vi "Shooter Control.vi"(11 "Time Delay Milli":u32) -> ()   [LabVIEW 2011]
uses:
  System Set Points and States.vi
  <vilib>/addons/control/pid/pid.llb/PID (DBL).vi
  <vilib>/addons/control/pid/NI_PID_pid.lvlib
panel:
  out "Stable":bool
  out "RPM Error":cluster{dbl, dbl, dbl[]}(graph)
  out "Output 2":dbl
  out "Output":dbl
  out "Shooter Enabled":bool
  in  "Graph time interval  in seconds":dbl
  out "Shooter RPM":cluster{dbl, dbl, dbl[]}(graph)
  out "RPM Error":dbl
  out "Encoder Speed":dbl
  in  "D":dbl
  in  "I":dbl=0.0068
  in  "P":dbl=0.0017 step=0.001
  out "Encoder Set Speed":dbl
  # "These Work\n0.0045\n0.05\n0.0005"
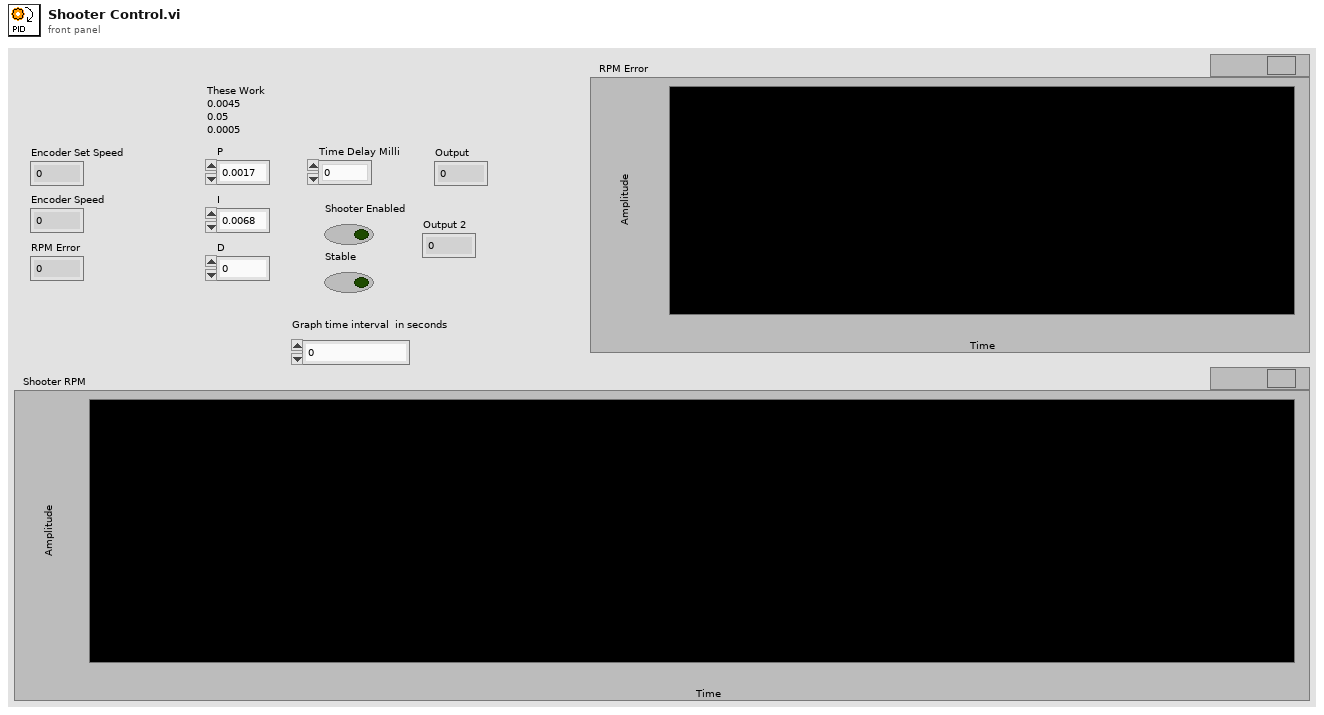
[diagram p1: front panel]
types:
  T1 = typedef "WPI_EncoderDevRef.ctl" = cluster{"DevStatus":errorcluster, "EncoderIndex":T2, "CounterIndex":T3, "DistancePerCount":dbl, "Decoding Type":T4}
  T2 = typedef "FPGA_EncoderIdx.ctl" = enum8{"Enc 0", "Enc 1", "Enc 2", "Enc 3", "Invalid"}
  T3 = typedef "FPGA_CounterCtrSystemIndex.ctl" = enum8{"Ctr 0", "Ctr 1", "Ctr 2", "Ctr 3", "Ctr 4", "Ctr 5", "Ctr 6", "Ctr 7", "Invalid"}
  T4 = typedef "WPI_EncoderType.ctl" = enum16{"1x", "2x", "4x"}
  T5 = typedef "WPI_MotorControlDeviceRef.ctl" = cluster{"DeviceStatus":errorcluster, "Type":enum16{"PWM", "CAN"}, "PWM":cluster{"Digital Module":T6, "PWM Channel":T7, "DeadBand":T8}, "CAN":cluster{"Device Number":u8, "Control Mode":T9, "Semaphore":T10, "Max Vout":dbl}, "Invert":bool, "TransformRef":T11, "InvTransformRef":T11}
  T6 = typedef "FPGA_TypedefDigitalModule.ctl" = enum16{"Digital Module 1", "Digital Module 2"}
  T7 = typedef "FPGA_DIOPWMChannel.ctl" = enum8{"PWM 1", "PWM 2", "PWM 3", "PWM 4", "PWM 5", "PWM 6", "PWM 7", "PWM 8", "PWM 9", "PWM 10", "Invalid"}
  T8 = typedef "WPI_PWMDeadband.ctl" = cluster{"Name":string, "maxPositivePwm":i32, "minPositivePwm":i32, "centerPwm":i32, "maxNegativePwm":i32, "minNegativePwm":i32, "angularRange":u16}
  T9 = typedef "WPI_CANJaguar_ControlMode.ctl" = enum8{"Percent VBus", "Current", "Speed", "Position", "Voltage"}
  T10 = typedef "Semaphore RefNum" = refnum<k1>
  T11 = typedef "WPI_PWMTransform_ConPane.ctl" = refnum<vi>
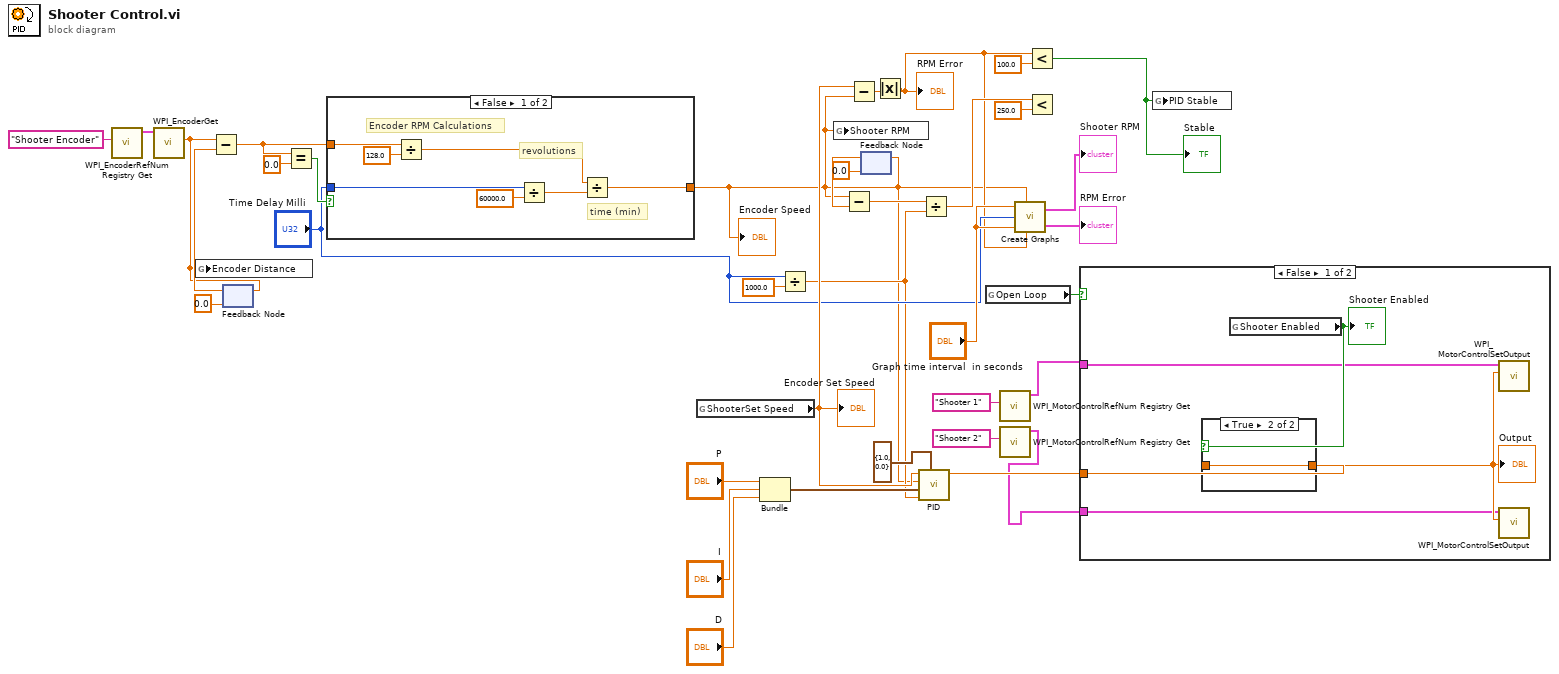
[diagram p0: block diagram]
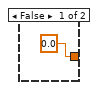
[diagram p2: hidden frame]
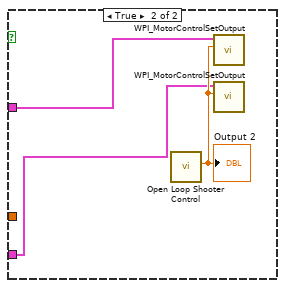
[diagram p3: hidden frame]
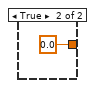
[diagram p4: hidden frame]
diagram:
  n1 = call <vilib>:"WPI_EncoderRefNum Registry Get.vi"("refnum name"="Shooter Encoder") -> ("EncoderDevRef"=w25:T1)  [unwired: 9 in, 1 out]
  n2 = call <vilib>:"WPI_EncoderGet.vi"("EncoderDevRef"=w25) -> ("Distance"=w21:dbl)  [unwired: 5 in, 5 out]
  n3 = global write "System Set Points and States.vi" "Encoder Distance"(w21) -> ()
  n4 = feedback #1(0.0) -> (w30:dbl)
  n5 = Subtract(x=w21, y=w30) -> (x-y=w22:dbl)
  n6 = feedback-in #1(w21) -> ()
  n7 = Equal?(x=w22, y=0.0) -> (x = y?=w27:bool)
  n8 = case shown="False" w27 {
    tunnel: [w43 0.0] -> w6
    tunnel: w22 -> [w42 _]
    tunnel: "Time Delay Milli" -> [w40 _]
    frame False {
      # "time (min)"
      # "revolutions"
      # "Encoder RPM Calculations"
      n9 = Divide(x=w42, y=128.0) -> (x/y=w41:dbl)
      n10 = Divide(x=w40, y=60000.0) -> (x/y=w38:dbl)
      n11 = Divide(x=w41, y=w38) -> (x/y=w43:dbl)
    }
    frame True {
    }
  }
  "Encoder Speed" <- w6
  n12 = global read "System Set Points and States.vi" "ShooterSet Speed"() -> (w31:dbl)
  "Encoder Set Speed" <- w31
  n13 = Bundle("P"="P", "I"="I", "D"="D") -> (w32:cluster{"P":dbl, "I":dbl, "D":dbl})  [unwired: 1 in]
  n14 = Divide(x="Time Delay Milli", y=1000.0) -> (x/y=w9:dbl)
  n15 = global write "System Set Points and States.vi" "Shooter RPM"(w6) -> ()
  n16 = Subtract(x=w31, y=w6) -> (x-y=w8:dbl)
  n17 = feedback-in #2(w6) -> ()
  n18 = feedback #2(0.0) -> (w20:dbl)
  n19 = Subtract(x=w6, y=w20) -> (x-y=w19:dbl)
  n20 = Absolute Value(x=w8) -> (abs(x)=w7:dbl)
  "RPM Error" <- w7
  n21 = call-poly <vilib>:"PID.vi"("output range"=cluster{"output high":dbl, "output low":dbl} {"output high"=1.0, "output low"=0.0}, "dt (s)"=w9, "PID gains"=w32, "process variable"=w6, "setpoint"=w31) -> ("output"=w24:dbl)  [unwired: 5 in, 1 out]
  n22 = Divide(x=w19, y=w9) -> (x/y=w18:dbl)
  n23 = global read "System Set Points and States.vi" "Open Loop"() -> (w23:bool)
  n24 = call <vilib>:"WPI_MotorControlRefNum Registry Get.vi"("refnum name"="Shooter 1") -> ("MotorControlDevRef"=w2:T5)  [unwired: 9 in, 1 out]
  n25 = call <vilib>:"WPI_MotorControlRefNum Registry Get.vi"("refnum name"="Shooter 2") -> ("MotorControlDevRef"=w1:T5)  [unwired: 9 in, 1 out]
  n26 = call "Create Graphs.vi"("Speed Graph Time"="Graph time interval  in seconds", "Speed"=w6, "Time Delay"="Time Delay Milli", "Error Graph Time"="Graph time interval  in seconds", "Error"=w7) -> ("Speed"=→"Shooter RPM":cluster{dbl, dbl, dbl[]}, "Error"=→"RPM Error":cluster{dbl, dbl, dbl[]})
  n27 = Less?(x=w7, y=100.0) -> (x < y?=w5:bool)
  "Stable" <- w5
  n28 = Less?(x=w18, y=250.0) -> ()  [unwired: 1 out]
  n29 = case shown="False" w23 {
    tunnel: w24 -> [w49 _]
    tunnel: w1 -> [w46 w52]
    tunnel: w2 -> [w45 w53]
    frame False {
      n30 = global read "System Set Points and States.vi" "Shooter Enabled"() -> (w48:bool)
      "Shooter Enabled" <- w48
      n31 = case shown="True" w48 {
        tunnel: w49 -> [_ w51]
        tunnel: [0.0 ("output") w51] -> w47
        frame False {
        }
        frame True {
        }
      }
      "Output" <- w47
      n32 = call <vilib>:"WPI_MotorControlSetOutput.vi"("Output"=w47, "MotorControlDevRef"=w45) -> ()  [unwired: 8 in, 2 out]
      n33 = call <vilib>:"WPI_MotorControlSetOutput.vi"("Output"=w47, "MotorControlDevRef"=w46) -> ()  [unwired: 8 in, 2 out]
    }
    frame True {
      n34 = call "Open Loop Shooter Control.vi"() -> ("Open Loop PWM"=w54:dbl)  [unwired: 11 in]
      "Output 2" <- w54
      n35 = call <vilib>:"WPI_MotorControlSetOutput.vi"("Output"=w54, "MotorControlDevRef"=w53) -> ()  [unwired: 8 in, 2 out]
      n36 = call <vilib>:"WPI_MotorControlSetOutput.vi"("Output"=w54, "MotorControlDevRef"=w52) -> ()  [unwired: 8 in, 2 out]
    }
  }
  n37 = global write "System Set Points and States.vi" "PID Stable"(w5) -> ()
